vi "PathPlanner_EventMarker_GetWaypointRelativePos.vi"(11 "in EventMarker":T1) -> (3 "WaypointRelativePos":dbl)   [LabVIEW 2019, in "PathPlanner24.lvlib"]
doc: "Get the waypoint relative position of this marker\n\nInputs:\n - EventMarker - cluster - Data cluster\n\nOutputs:\n - WaypointRelativePose - double - The waypoint relative position of the marker"
uses:
  PathPlanner24.lvlib
  TypeDef/PathPlannerEventMarker.ctl
  TypeDef/PathPlannerCommandUtil.ctl
  ENum/PathPlanner_CommandUtil_Type_ENUM.ctl
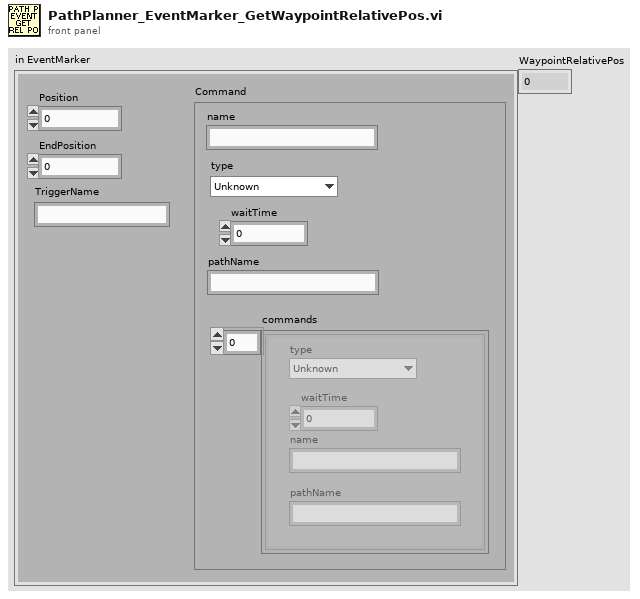
[diagram p1: front panel]
types:
  T1 = typedef "PathPlanner24.lvlib/PathPlannerEventMarker.ctl" = cluster{"Position":dbl, "Command":T2, "TriggerName":string, "EndPosition":dbl}
  T2 = typedef "PathPlanner24.lvlib/PathPlannerCommandUtil.ctl" = cluster{"waitTime":dbl, "name":string, "pathName":string, "commands":cluster{"type":T3, "waitTime":dbl, "name":string, "pathName":string}[], "type":T3}
  T3 = typedef "PathPlanner24.lvlib/PathPlanner_CommandUtil_Type_ENUM.ctl" = enum16{"Unknown", "Wait", "Named", "Path", "Sequential", "Parallel", "Race", "Deadline"}
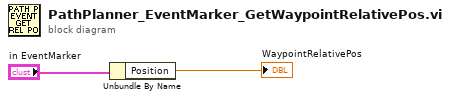
[diagram p0: block diagram]
diagram:
  n1 = Unbundle By Name("in EventMarker") -> ("Position"=→"WaypointRelativePos":dbl)
